vi "macro_BoolCmd_Recv.vi"() -> ()   [LabVIEW 2019, in "Trajectory_Library.lvlib"]
uses:
  VI/DigSeqLogic_Edge_On.vi
  VI/BoolCmd_Send_Internal.vi
  VI/BoolCmd_ObtainQueue.vi
  Trajectory_Library.lvlib
panel:
  out "New Request":bool
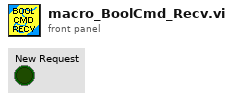
[diagram p1: front panel]
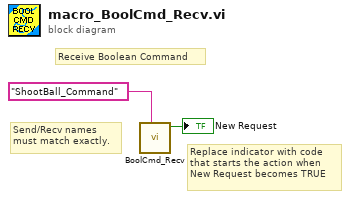
[diagram p0: block diagram]
diagram:
  # "Send/Recv names\nmust match exactly."
  # "Replace indicator with code\nthat starts the action when \nNew Request becomes TRUE"
  # "Receive Boolean Command"
  n1 = call "BoolCmd_Recv.vi"("Command Name"="ShootBall_Command") -> ("New Request"=→"New Request":bool)  [unwired: 9 in, 1 out]
